vi "Read IBW File.vi"(8 "error in (no error)":errorcluster, 10 "Basename":string, 11 "Path":path) -> (0 "error out":errorcluster, 2 "Notes LUT":variant, 3 "IMAQ":T1[](array[plugin-control]))   [LabVIEW 2019]
uses:
  <vilib>/vision/NI_Vision_Development_Module.lvlib
  <vilib>/Utility/error.llb/whitespace.ctl
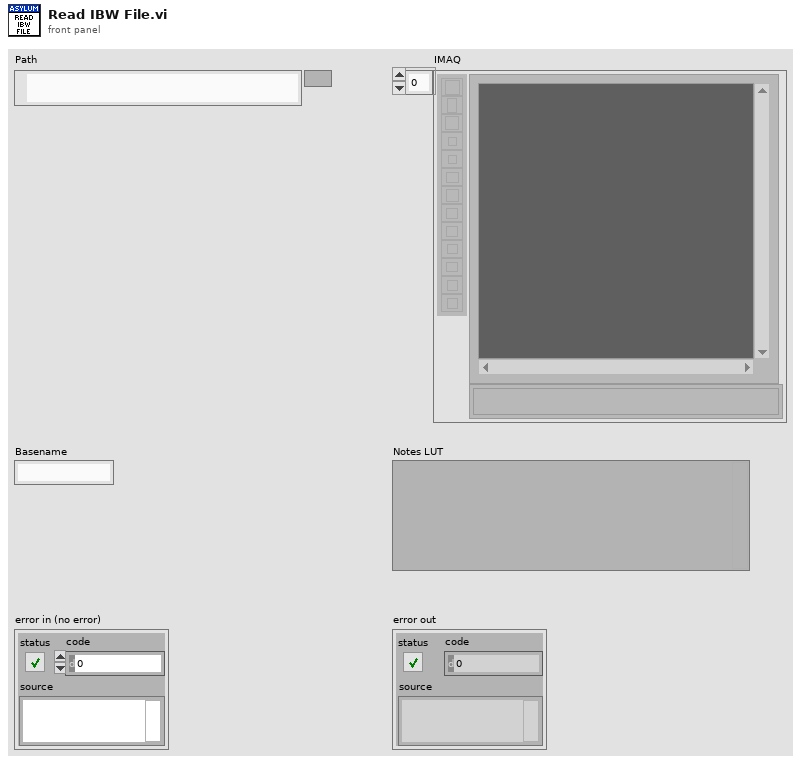
[diagram p1: front panel]
types:
  T1 = typedef "IMAQ Image.ctl" = refnum<image>
  T2 = enum32{"Invalid", "Standard", "Closed", "Hidden", "Minimized", "Maximized"}
  T3 = enum32{"invalid app kind", "Development System", "Run Time System", "Student Edition", "Embedded LabVIEW", "Evaluation", "Custom"}
  T4 = enum16{"big-endian, network order", "native, host order", "little-endian"}
  T5 = cluster{"Core":cluster{"Current VI Reference":refnum<vi>, "Close Panel on Exit?":bool}, "Binary":string, "wfmSize":i32, "noteSize":i32, "nDim":i32[], "wData":sgl[], "Shaped wData":sgl[][][], "Notes":string}
  T6 = cluster{"Current VI Reference":refnum<vi>, "Close Panel on Exit?":bool}
  T7 = typedef "Image Type" = u32
  T8 = typedef "whitespace.ctl" = u16
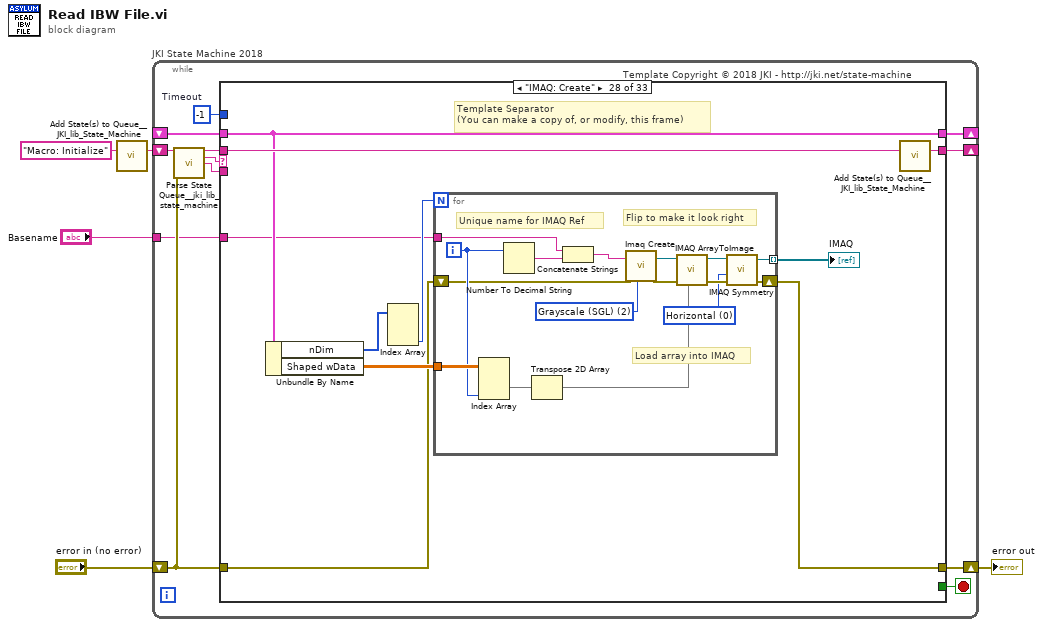
[diagram p0: block diagram]
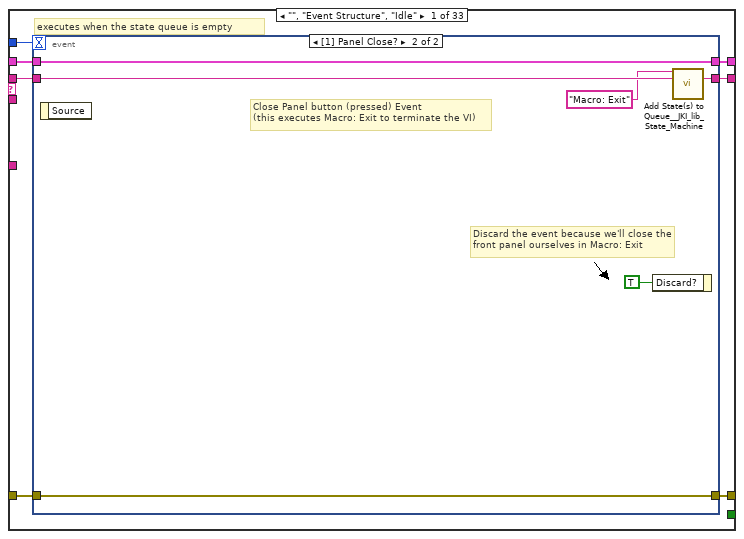
[diagram p2: hidden frame]
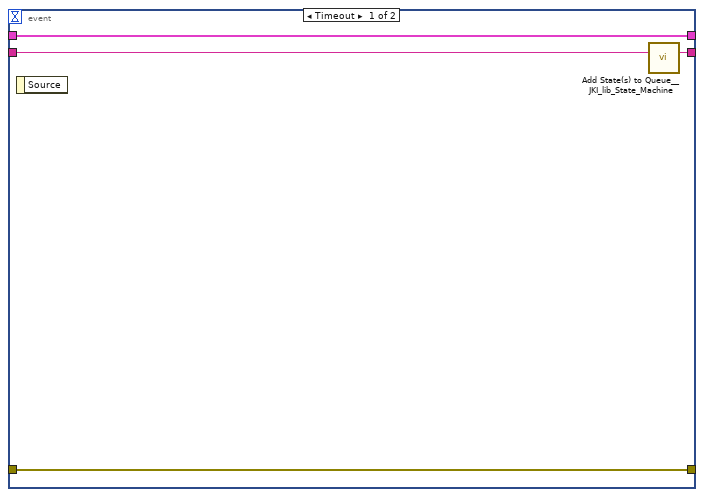
[diagram p3: hidden frame]
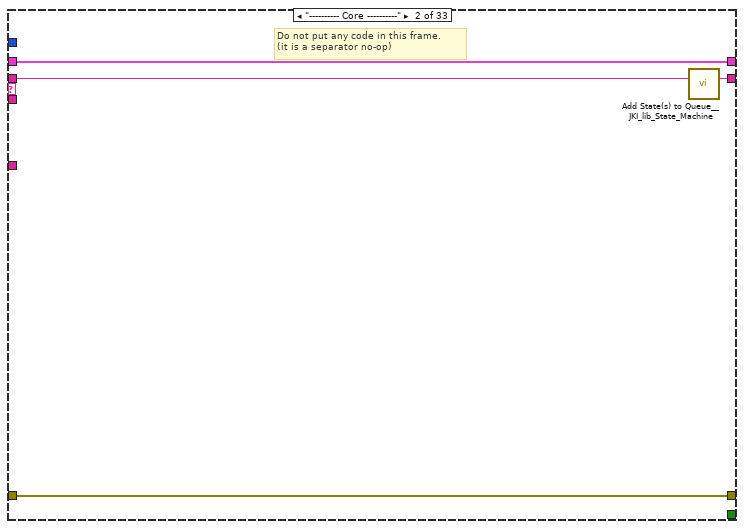
[diagram p4: hidden frame]
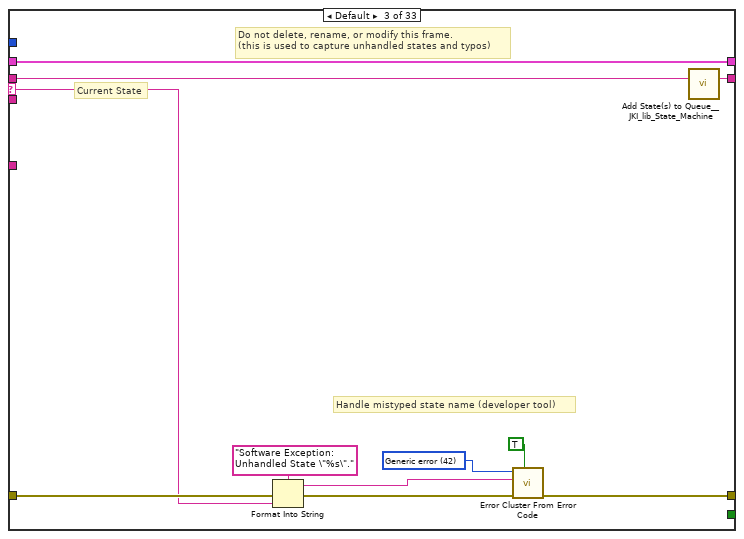
[diagram p5: hidden frame]
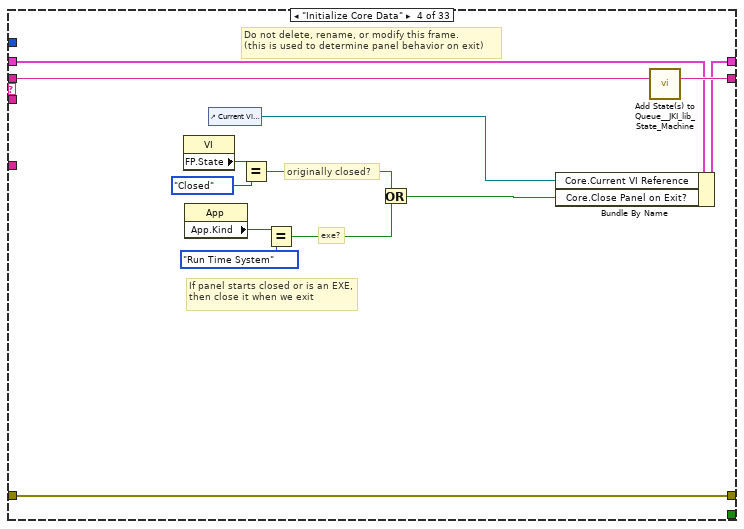
[diagram p6: hidden frame]
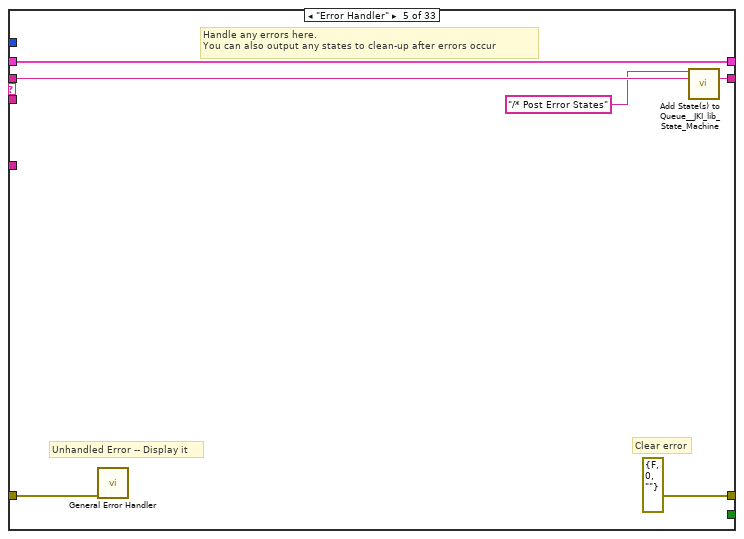
[diagram p7: hidden frame]
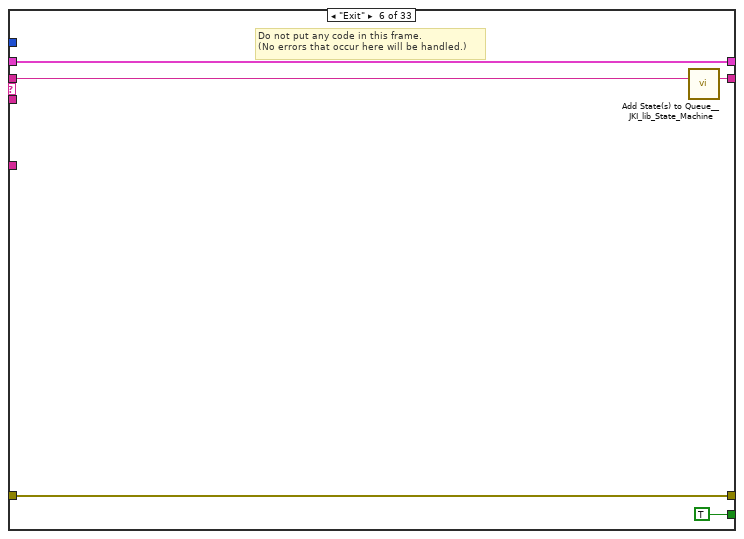
[diagram p8: hidden frame]
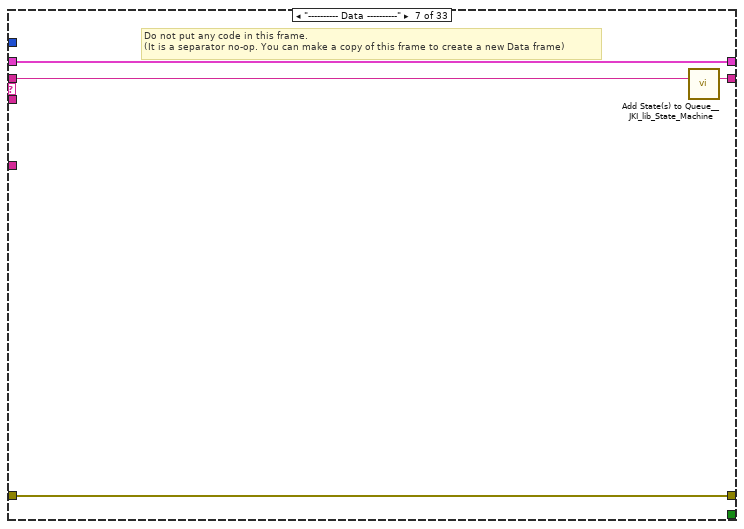
[diagram p9: hidden frame]
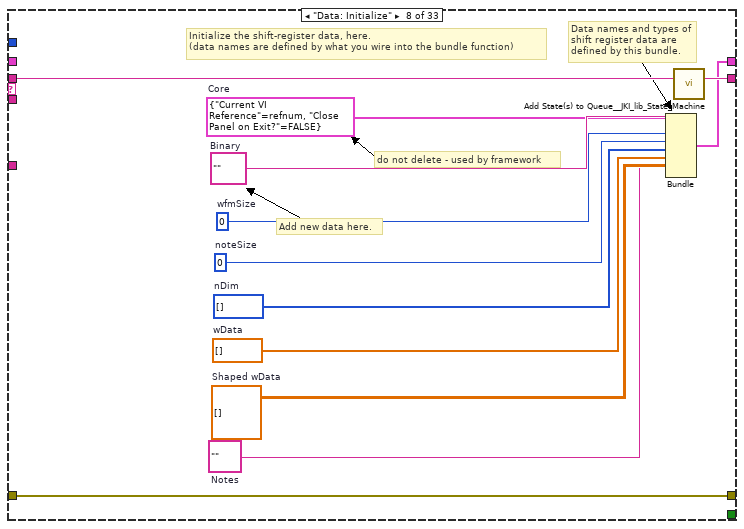
[diagram p10: hidden frame]
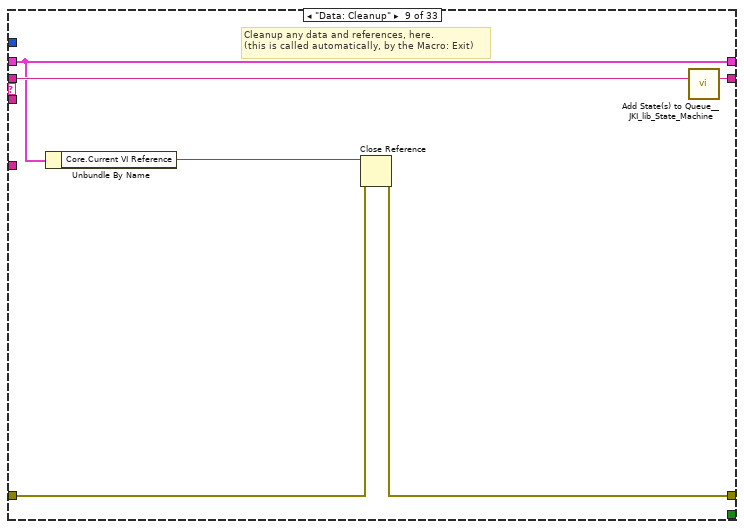
[diagram p11: hidden frame]
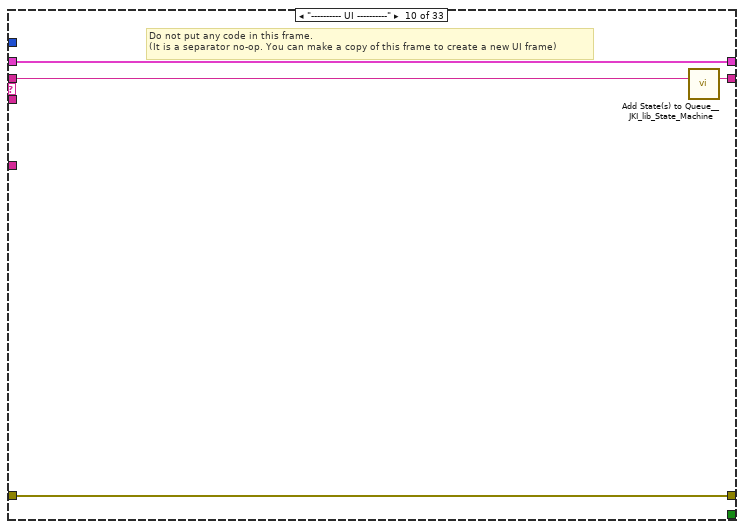
[diagram p12: hidden frame]
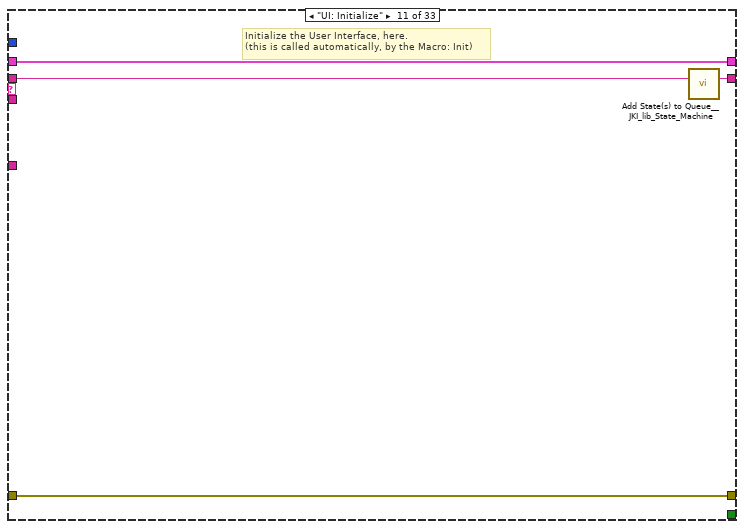
[diagram p13: hidden frame]
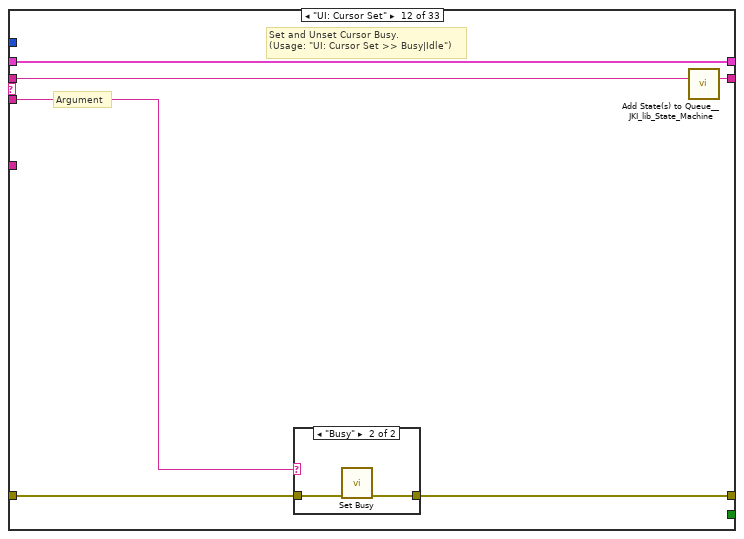
[diagram p14: hidden frame]
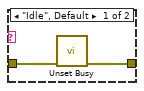
[diagram p15: hidden frame]
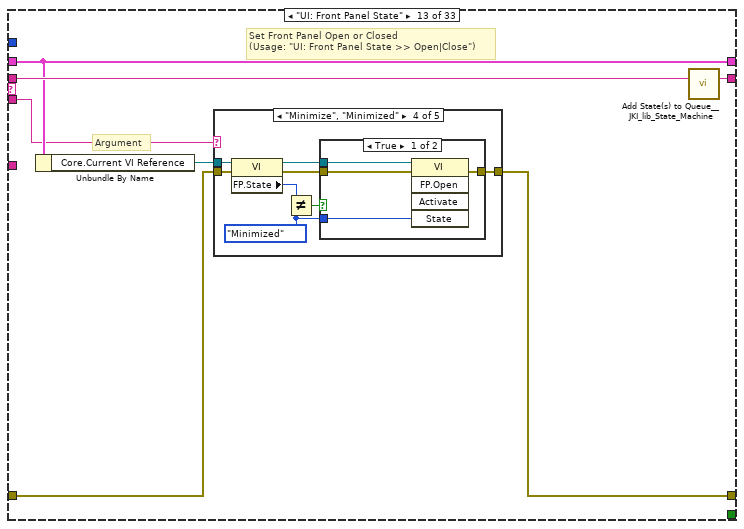
[diagram p16: hidden frame]
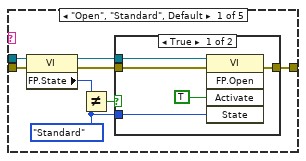
[diagram p17: hidden frame]
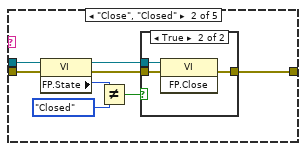
[diagram p19: hidden frame]
diagram:
  n1 = call <vilib>:"Add State(s) to Queue__JKI_lib_State_Machine.vi"("State(s) in (\"\")"="Macro: Initialize") -> ("States Out"=w5:string)  [unwired: 14 in]
  n2 = while "JKI State Machine 2018" {
    shift-right: [w10] -> _
    shift-left: _ -> [w9]
    shift-right: [w13] -> w3
    shift-left: "error in (no error)" -> [w7]
    shift-right: [w12] -> _
    shift-left: w5 -> [w14]
    tunnel: "Basename" -> [w6]
    stop <- w11 stop-if-true
    w8 = -1  # Timeout
    # "Template Copyright © 2018 JKI - http://jki.net/state-machine"
    n3 = call <vilib>:"Parse State Queue__jki_lib_state_machine.vi"("State Queue"=w14, "Error In (no error)"=w7) -> ("Remaining States"=w16:string, "Current State"=w17:string, "Arguments"=w15:string)  [unwired: 11 in]
    n4 = case shown="\"IMAQ: Create\"" w17 {
      selector: w17 -> [_ _ w39 _ _ _ _ _ _ _ _ _ _ _ _ _ _ _ _ _ _ _ _ _ _ _ _ _ _ _ _ _ _]
      tunnel: w16 -> [w24 w38 w43 w62 w68 w73 w77 w89 w95 w99 w103 w109 w120 w189 w194 w199 w209 w213 w221 w225 w238 w251 w264 w285 w300 w336 w340 w350 w370 w380 w403 w407 w411]
      tunnel: w15 -> [_ _ _ _ _ _ _ _ _ _ _ w104 w114 _ _ _ _ _ _ _ _ _ _ _ _ _ _ _ _ _ _ _ _]
      tunnel: w9 -> [w22 w35 w41 w55 w65 w71 w74 _ w90 w96 w101 w107 w116 w186 w191 w196 w206 w210 w217 w222 w227 w240 w254 w275 w292 w327 w337 w343 w367 w378 w400 w404 w408]
      tunnel: [w21 w36 w45 w59 errorcluster {"status"=FALSE, "code"=0, "source"=""} ("error out") w70 w75 w86 w91 w97 w100 w105 w117 w187 w192 w197 w207 w211 w215 w223 w236 w249 w262 w266 w298 w334 w338 w344 w368 w372 w401 w405 w409] -> w13
      tunnel: w7 -> [w20 w36 w44 w59 w64 w70 w75 w86 w92 w97 w100 w106 w118 w187 w192 w197 w207 w211 w214 w223 w236 w249 w262 w267 w298 w334 w338 w345 w368 w371 w401 w405 w409]
      tunnel: [w23 w37 w42 w61 w67 w72 w76 w88 w94 w98 w102 w108 w119 w188 w193 w198 w208 w212 w220 w224 w237 w250 w263 w284 w299 w335 w339 w349 w369 w379 w402 w406 w410] -> w12
      tunnel: [_ _ _ _ _ TRUE _ _ _ _ _ _ _ _ _ _ _ _ _ _ _ _ _ _ _ _ _ _ _ _ _ _ _] -> w11
      tunnel: [w19 w35 w41 w60 w65 w71 w74 w87 w90 w96 w101 w107 w116 w186 w191 w196 w206 w210 w218 w222 w228 w241 w255 w276 w293 w328 w337 w343 w367 w378 w400 w404 w408] -> w10
      tunnel: w8 -> [w18 _ _ _ _ _ _ _ _ _ _ _ _ _ _ _ _ _ _ _ _ _ _ _ _ _ _ _ _ _ _ _ _]
      tunnel: w6 -> [_ _ _ _ _ _ _ _ _ _ _ _ _ _ _ _ _ _ _ _ _ _ _ _ _ _ _ w342 _ _ _ _ _]
      frame "", "Event Structure", "Idle" {
        # "executes when the state queue is empty"
        n5 = event shown="[1] Panel Close?" {
          selector: _ -> [_ _]
          dyn-events: _ -> [_ _]
          timeout: w18 -> [_ _]
          tunnel: w24 -> [w28 w34]
          tunnel: [w27 w33] -> w23
          tunnel: w22 -> [w25 w31]
          tunnel: [w26 w32] -> w21
          tunnel: w20 -> [w26 w32]
          tunnel: [w25 w31] -> w19
          event Timeout {
            n6 = event-data() -> ()  [unwired: 1 in, 1 out]
            n7 = call <vilib>:"Add State(s) to Queue__JKI_lib_State_Machine.vi"("State(s) in (\"\")"=w28) -> ("States Out"=w27:string)  [unwired: 14 in]
          }
          event Panel Close? {
            # "Discard the event because we'll close the front panel ourselves in Macro: Exit"
            # "Close Panel button (pressed) Event\n(this executes Macro: Exit to terminate the VI)"
            n8 = event-data() -> ()  [unwired: 1 in, 1 out]
            n9 = event-data ("Event Filter Node")("Discard?"=TRUE) -> ()  [unwired: 1 in, 1 out]
            n10 = call <vilib>:"Add State(s) to Queue__JKI_lib_State_Machine.vi"("State(s) in Front (\"\")"="Macro: Exit", "State(s) in (\"\")"=w34) -> ("States Out"=w33:string)  [unwired: 13 in]
          }
        }
      }
      frame "---------- Core ----------" {
        # "Do not put any code in this frame.\n(it is a separator no-op)"
        n11 = call <vilib>:"Add State(s) to Queue__JKI_lib_State_Machine.vi"("State(s) in (\"\")"=w38) -> ("States Out"=w37:string)  [unwired: 14 in]
      }
      frame Default {
        w48 = 42 items=["No error", "Argument error", "Memory is full", "Out of zone", "End of file", "File already open", "Generic file I/O error", "File not found", "File permission error", "Disk is full", "Duplicate path", "Too many files open", "System feature not enabled", "Resource file not found", "Cannot add resource", "Resource not found", "Image not found", "Image memory error", "Pen does not exist", "Config type invalid", "Config token not found", "Config parse error", "Config memory error", "Bad external code format", "Bad external code offset", "External code not present", "Null window", "Destroy window error", "Null menu", "Print aborted", "Bad print record", "Print driver error", "Windows error during printing", "Memory error during printing", "Print dialog error", "Generic print error", "Invalid device refnum", "Device not found", "Device parameter error", "Device unit error", "Cannot open device", "Device call aborted", "Generic error", "Cancelled by user", "Object ID too low", "Object ID too high", "Object not in heap", "Unknown heap", "Unknown object (invalid DefProc)", "Unknown object (DefProc not in table)", "Message out of range", "Invalid (null) method", "Unknown message", "Manager call not supported", "Bad address", "Network operation in progress", "Network operation timed out", "Connection is busy", "Network attribute not supported", "Network error", "Address in use", "System out of memory", "Connection aborted", "Connection refused", "Not connected", "Already connected", "Connection closed", "Initialization error (interapplication manager)", "Bad occurrence", "Wait on unbound occurrence handler", "Occurrence queue overflow", "Datalog type conflict", "Unused", "Unrecognized type (interapplication manager)", "Memory corrupt", "Failed to make temporary DLL", "Old CIN version", "Drag socket not found", "Failed to load drop-object", "Failed to register OLE object", "Failed to release OLE object", "Format specifier type mismatch", "Unknown format specifier", "Too few format specifiers", "Too many format specifiers", "Scan failed", "Newer CIN version", "Error converting to variant", "Runtime menu error", "Password tampered", "Variant attribute not found", "Incompatible variant data type", "Event data is not available", "Event Store is not present", "Occurrence is not found", "Event Queue is not created", "Event info is not available", "Refnum passed is NULL", "Error retrieving Class GUID", "Error retrieving CoClass GUID", "Error retrieving TypeLib GUID.", "Bad built application magic bytes.", "Specific driver is different from the specific driver associated with the Logical Name.", "There is no session opened to the class driver.", "Max Error", "MAX - Error with config objects", "MAX - Error loading configuration", "MAX - Group not supported"]
        # "Current State"
        # "Do not delete, rename, or modify this frame.\n(this is used to capture unhandled states and typos)"
        # "Handle mistyped state name (developer tool)"
        n12 = Format Into String(format string="Software Exception: Unhandled State \"%s\"." ("message"), error in=w44, w39) -> (resulting string=w47:string, error out=w46:errorcluster)  [unwired: 1 in]
        n13 = call <vilib>:"Error Cluster From Error Code.vi"("show call chain? (False)"=TRUE, "error in (no error)"=w46, "error message (\"\")"=w47, "error code (0)"=w48) -> ("error out"=w45:errorcluster)  [unwired: 5 in]
        n14 = call <vilib>:"Add State(s) to Queue__JKI_lib_State_Machine.vi"("State(s) in (\"\")"=w43) -> ("States Out"=w42:string)  [unwired: 14 in]
      }
      frame "Initialize Core Data" {
        # "Do not delete, rename, or modify this frame.\n(this is used to determine panel behavior on exit)"
        # "originally closed?"
        # "exe?"
        # "If panel starts closed or is an EXE, then close it when we exit"
        n15 = property on="Property Node" class="VI"() -> ("FP.State"=w52:T2)  [unwired: 2 in, 2 out]
        n16 = property on="Property Node" class="App"() -> ("App.Kind"=w58:T3)  [unwired: 2 in, 2 out]
        n17 = control-ref of="Current VI Reference"() -> (w53:refnum<vi>)
        n18 = Equal?(x=w52, y=T2."Closed" ("Front Panel Window:State")) -> (x = y?=w50:bool)
        n19 = Equal?(x=w58, y=T3."Run Time System" ("Application:Kind")) -> (x = y?=w56:bool)
        n20 = Or(x=w50, y=w56) -> (x .or. y?=w54:bool)
        n21 = Bundle By Name(cluster=w55, "Core.Current VI Reference"=w53, "Core.Close Panel on Exit?"=w54) -> (w60:T5)
        n22 = call <vilib>:"Add State(s) to Queue__JKI_lib_State_Machine.vi"("State(s) in (\"\")"=w62) -> ("States Out"=w61:string)  [unwired: 14 in]
      }
      frame "Error Handler" {
        # "Unhandled Error -- Display it"
        # "Handle any errors here.\nYou can also output any states to clean-up after errors occur"
        # "Clear error"
        n23 = call <vilib>:"General Error Handler.vi"("error in (no error)"=w64) -> ()  [unwired: 10 in, 5 out]
        n24 = call <vilib>:"Add State(s) to Queue__JKI_lib_State_Machine.vi"("State(s) in Front (\"\")"="/* Post Error States", "State(s) in (\"\")"=w68) -> ("States Out"=w67:string)  [unwired: 13 in]
      }
      frame "Exit" {
        # "Do not put any code in this frame.\n(No errors that occur here will be handled.)"
        n25 = call <vilib>:"Add State(s) to Queue__JKI_lib_State_Machine.vi"("State(s) in (\"\")"=w73) -> ("States Out"=w72:string)  [unwired: 14 in]
      }
      frame "---------- Data ----------" {
        # "Do not put any code in this frame.\n(It is a separator no-op. You can make a copy of this frame to create a new Data frame)"
        n26 = call <vilib>:"Add State(s) to Queue__JKI_lib_State_Machine.vi"("State(s) in (\"\")"=w77) -> ("States Out"=w76:string)  [unwired: 14 in]
      }
      frame "Data: Initialize" {
        w78 = ""  # Notes
        w79 = sgl[][][] []  # Shaped wData
        w80 = sgl[] []  # wData
        w81 = i32[] []  # nDim
        w82 = 0  # noteSize
        w83 = 0  # wfmSize
        w84 = T6 {"Current VI Reference"=refnum, "Close Panel on Exit?"=FALSE}  # Core
        w85 = ""  # Binary
        # "do not delete - used by framework"
        # "Add new data here."
        # "Data names and types of shift register data are defined by this bundle."
        # "Initialize the shift-register data, here.\n(data names are defined by what you wire into the bundle function)"
        n27 = Bundle("Core"=w84, "Binary"=w85, "wfmSize"=w83, "noteSize"=w82, "nDim"=w81, "wData"=w80, "Shaped wData"=w79, "Notes"=w78) -> (w87:T5)  [unwired: 1 in]
        n28 = call <vilib>:"Add State(s) to Queue__JKI_lib_State_Machine.vi"("State(s) in (\"\")"=w89) -> ("States Out"=w88:string)  [unwired: 14 in]
      }
      frame "Data: Cleanup" {
        # "Cleanup any data and references, here.\n(this is called automatically, by the Macro: Exit)"
        n29 = Unbundle By Name(w90) -> ("Core.Current VI Reference"=w93:refnum<vi>)
        n30 = Close Reference(reference=w93, error in (no error)=w92) -> (error out=w91:errorcluster)
        n31 = call <vilib>:"Add State(s) to Queue__JKI_lib_State_Machine.vi"("State(s) in (\"\")"=w95) -> ("States Out"=w94:string)  [unwired: 14 in]
      }
      frame "---------- UI ----------" {
        # "Do not put any code in this frame.\n(It is a separator no-op. You can make a copy of this frame to create a new UI frame)"
        n32 = call <vilib>:"Add State(s) to Queue__JKI_lib_State_Machine.vi"("State(s) in (\"\")"=w99) -> ("States Out"=w98:string)  [unwired: 14 in]
      }
      frame "UI: Initialize" {
        # "Initialize the User Interface, here.\n(this is called automatically, by the Macro: Init)"
        n33 = call <vilib>:"Add State(s) to Queue__JKI_lib_State_Machine.vi"("State(s) in (\"\")"=w103) -> ("States Out"=w102:string)  [unwired: 14 in]
      }
      frame "UI: Cursor Set" {
        # "Argument"
        # "Set and Unset Cursor Busy.\n(Usage: \"UI: Cursor Set >> Busy|Idle\")"
        n34 = case shown="\"Busy\"" w104 {
          tunnel: w106 -> [w111 w113]
          tunnel: [w110 w112] -> w105
          frame "Idle", Default {
            n35 = call <vilib>:"Unset Busy.vi"("error in (no error)"=w111) -> ("error out"=w110:errorcluster)  [unwired: 10 in]
          }
          frame "Busy" {
            n36 = call <vilib>:"Set Busy.vi"("error in (no error)"=w113) -> ("error out"=w112:errorcluster)  [unwired: 9 in, 1 out]
          }
        }
        n37 = call <vilib>:"Add State(s) to Queue__JKI_lib_State_Machine.vi"("State(s) in (\"\")"=w109) -> ("States Out"=w108:string)  [unwired: 14 in]
      }
      frame "UI: Front Panel State" {
        # "Argument"
        # "Set Front Panel Open or Closed\n(Usage: \"UI: Front Panel State >> Open|Close\")"
        n38 = Unbundle By Name(w116) -> ("Core.Current VI Reference"=w115:refnum<vi>)
        n39 = case shown="\"Minimize\", \"Minimized\"" w114 {
          tunnel: w118 -> [w126 w141 w152 w165 w178]
          tunnel: [w128 w142 w154 w167 w180] -> w117
          tunnel: w115 -> [w127 w139 w153 w166 w179]
          frame "Open", "Standard", Default {
            w121 = T2."Standard" ("State")
            n40 = property on="Property Node" class="VI"(reference=w127, error in=w126) -> (reference out=w124:refnum<vi>, error out=w125:errorcluster, "FP.State"=w123:T2)
            n41 = Not Equal?(x=w123, y=w121) -> (x != y?=w122:bool)
            n42 = case shown="True" w122 {
              tunnel: [w132 w134] -> w128
              tunnel: w125 -> [w131 w134]
              tunnel: w124 -> [w130 _]
              tunnel: w121 -> [w129 _]
              frame True {
                n43 = invoke on="Invoke Node" class="VI" method="FP.Open"(reference=w130, error in=w131, "Activate"=TRUE, "State"=w129) -> (error out=w132:errorcluster)  [unwired: 1 in, 4 out]
              }
              frame False {
              }
            }
          }
          frame "Close", "Closed" {
            n44 = property on="Property Node" class="VI"(reference=w139, error in=w141) -> (reference out=w138:refnum<vi>, error out=w140:errorcluster, "FP.State"=w136:T2)
            n45 = Not Equal?(x=w136, y=T2."Closed" ("Front Panel Window:State")) -> (x != y?=w135:bool)
            n46 = case shown="True" w135 {
              tunnel: [w143 w146] -> w142
              tunnel: w140 -> [w143 w145]
              tunnel: w138 -> [_ w144]
              frame False {
              }
              frame True {
                n47 = invoke on="Invoke Node" class="VI" method="FP.Close"(reference=w144, error in=w145) -> (error out=w146:errorcluster)  [unwired: 1 in, 2 out]
              }
            }
          }
          frame "Hidden", "Hide" {
            w147 = T2."Hidden" ("State")
            n48 = property on="Property Node" class="VI"(reference=w153, error in=w152) -> (reference out=w150:refnum<vi>, error out=w151:errorcluster, "FP.State"=w149:T2)
            n49 = Not Equal?(x=w149, y=w147) -> (x != y?=w148:bool)
            n50 = case shown="True" w148 {
              tunnel: [w158 w159] -> w154
              tunnel: w151 -> [w157 w159]
              tunnel: w150 -> [w156 _]
              tunnel: w147 -> [w155 _]
              frame True {
                n51 = invoke on="Invoke Node" class="VI" method="FP.Open"(reference=w156, error in=w157, "State"=w155) -> (error out=w158:errorcluster)  [unwired: 2 in, 4 out]
              }
              frame False {
              }
            }
          }
          frame "Minimize", "Minimized" {
            w160 = T2."Minimized" ("State")
            n52 = property on="Property Node" class="VI"(reference=w166, error in=w165) -> (reference out=w163:refnum<vi>, error out=w164:errorcluster, "FP.State"=w162:T2)
            n53 = Not Equal?(x=w162, y=w160) -> (x != y?=w161:bool)
            n54 = case shown="True" w161 {
              tunnel: [w171 w172] -> w167
              tunnel: w164 -> [w170 w172]
              tunnel: w163 -> [w169 _]
              tunnel: w160 -> [w168 _]
              frame True {
                n55 = invoke on="Invoke Node" class="VI" method="FP.Open"(reference=w169, error in=w170, "State"=w168) -> (error out=w171:errorcluster)  [unwired: 2 in, 4 out]
              }
              frame False {
              }
            }
          }
          frame "Maximize", "Maximized" {
            w173 = T2."Maximized" ("State")
            n56 = property on="Property Node" class="VI"(reference=w179, error in=w178) -> (reference out=w176:refnum<vi>, error out=w177:errorcluster, "FP.State"=w175:T2)
            n57 = Not Equal?(x=w175, y=w173) -> (x != y?=w174:bool)
            n58 = case shown="True" w174 {
              tunnel: [w184 w185] -> w180
              tunnel: w177 -> [w183 w185]
              tunnel: w176 -> [w182 _]
              tunnel: w173 -> [w181 _]
              frame True {
                n59 = invoke on="Invoke Node" class="VI" method="FP.Open"(reference=w182, error in=w183, "State"=w181) -> (error out=w184:errorcluster)  [unwired: 2 in, 4 out]
              }
              frame False {
              }
            }
          }
        }
        n60 = call <vilib>:"Add State(s) to Queue__JKI_lib_State_Machine.vi"("State(s) in (\"\")"=w120) -> ("States Out"=w119:string)  [unwired: 14 in]
      }
      frame "---------- Macro ----------" {
        # "Backups in case Directory State gets deleted on accident since those are never called"
        # "Length|Index|typedef struct BinHeader5 {\n     2|    0|\tshort version;\t\t\t\t\t\t          // Version number for backwards compatibility.\n     2|    2|\tshort checksum;\t\t\t\t\t\t         // Checksum over this header and the wave header.\n     4|    4|\tlong wfmSize;\t\t\t\t\t\t           // The size of the WaveHeader5 data structure plus the wave data.\n     4|    8|\tlong formulaSize;\t\t\t\t\t        // The size of the dependency formula, if any.\n     4|   12|\tlong noteSize;\t\t\t\t\t\t          // The size of the note text.\n     4|   16|\tlong dataEUnitsSize;\t\t\t\t      // The size of optional extended data units.\n    16|   20|\tlong dimEUnitsSize[MAXDIMS];\t\t// The size of optional extended dimension units.\n    16|   36|\tlong dimLabelsSize[MAXDIMS];\t\t// The size of optional dimension labels.\n     4|   52|\tlong sIndicesSize;\t\t\t\t\t       // The size of string indicies if this is a text wave.\n     4|   56|\tlong optionsSize1;\t\t\t\t\t       // Reserved. Write zero. Ignore on read.\n     4|   60|\tlong optionsSize2;\t\t\t\t\t       // Reserved. Write zero. Ignore on read.\n      |   64|} BinHeader5;"
        # "Length|Index|struct WaveHeader5 {\n     4|   64|\tstruct WaveHeader5 **next;\t\t\t  // link to next wave in linked list.\n     4|   68|\tunsigned long creationDate;\t\t \t// DateTime of creation.\n     4|   72|\tunsigned long modDate;\t\t\t\t     // DateTime of last modification.\n     4|   76|\tlong npnts;\t\t\t\t\t\t\t             // Total number of points (multiply dimensions up to first zero).\n     2|   80|\tshort type;\t\t\t\t\t\t\t             // See types (e.g. NT_FP64) above. Zero for text waves.\n     2|   82|\tshort dLock;\t\t\t\t\t\t             // Reserved. Write zero. Ignore on read.\n     6|   84|\tchar whpad1[6];\t\t\t\t\t\t          // Reserved. Write zero. Ignore on read.\n     2|   90|\tshort whVersion;\t\t\t\t\t          // Write 1. Ignore on read.\n    32|   92|\tchar bname[MAX_WAVE_NAME5+1];\t\t// Name of wave plus trailing null.\n     4|  124|\tlong whpad2;\t\t\t\t\t\t             // Reserved. Write zero. Ignore on read.\n     4|  128|\tstruct DataFolder **dFolder;\t\t // Used in memory only. Write zero. Ignore on read.\n      |     |\t// Dimensioning info. [0] == rows, [1] == cols etc\n    16|  132|\tlong nDim[MAXDIMS];\t\t\t\t\t       // Number of of items in a dimension -- 0 means no data.\n    32|  148|\tdouble sfA[MAXDIMS];\t\t\t\t       // Index value for element e of dimension d = sfA[d]*e + sfB[d].\n    32|  180|\tdouble sfB[MAXDIMS];\n      |     |\t// SI units\n     4|  212|\tchar dataUnits[MAX_UNIT_CHARS+1];\t\t\t      // Natural data units go here - null if none.\n    16|  216|\tchar dimUnits[MAXDIMS][MAX_UNIT_CHARS+1];\t// Natural dimension units go here - null if none.\n     2|  232|\tshort fsValid;\t\t\t\t\t\t                      // TRUE if full scale values have meaning.\n     2|  234|\tshort whpad3;\t\t\t\t\t\t                       // Reserved. Write zero. Ignore on read.\n    16|  236|\tdouble topFullScale,botFullScale;\t        // The max and max full scale value for wave.\n     4|  252|\tHandle dataEUnits;\t\t\t\t\t                   // Used in memory only. Write zero. Ignore on read.\n    16|  256|\tHandle dimEUnits[MAXDIMS];\t\t\t             // Used in memory only. Write zero. Ignore on read.\n    16|  272|\tHandle dimLabels[MAXDIMS];\t\t\t             // Used in memory only. Write zero. Ignore on read.\n     4|  288|\tHandle waveNoteH;\t\t\t\t\t                    // Used in memory only. Write zero. Ignore on read.\n    64|  292|\tlong whUnused[16];\t\t\t\t\t                   // Reserved. Write zero. Ignore on read.\n      |     |\t// The following stuff is considered private to Igor.\n     2|  356|\tshort aModified;\t\t\t\t\t                     // Used in memory only. Write zero. Ignore on read.\n     2|  358|\tshort wModified;\t\t\t\t\t                     // Used in memory only. Write zero. Ignore on read.\n     2|  360|\tshort swModified;\t\t\t\t\t                    // Used in memory only. Write zero. Ignore on read.\n     1|  362|\tchar useBits;\t\t\t\t\t\t                       // Used in memory only. Write zero. Ignore on read.\n     1|  363|\tchar kindBits;\t\t\t\t\t\t                      // Reserved. Write zero. Ignore on read.\n     4|  364|\tvoid **formula;\t\t\t\t\t\t                     // Used in memory only. Write zero. Ignore on read.\n     4|  368|\tlong depID;\t\t\t\t\t\t\t                        // Used in memory only. Write zero. Ignore on read.\n     2|  372|\tshort whpad4;\t\t\t\t\t\t                       // Reserved. Write zero. Ignore on read.\n     2|  374|\tshort srcFldr;\t\t\t\t\t\t                      // Used in memory only. Write zero. Ignore on read.\n     4|  376|\tHandle fileName;\t\t\t\t\t                     // Used in memory only. Write zero. Ignore on read.\n     4|  380|\tlong **sIndices;\t\t\t\t\t                     // Used in memory only. Write zero. Ignore on read.\n     4|  384|\tfloat wData[1];\t\t\t\t\t\t                     // The start of the array of data. Must be 64 bit aligned.\n      |  388|};"
        # "Do not put any code in this frame.\n(It is a separator no-op. You can make a copy of this frame to create a new Macro frame)"
        n61 = call <vilib>:"Add State(s) to Queue__JKI_lib_State_Machine.vi"("State(s) in (\"\")"=w189) -> ("States Out"=w188:string)  [unwired: 14 in]
      }
      frame "Macro: Initialize" {
        # "Initialization Macro\n(This is called once, when the VI starts)"
        n62 = call <vilib>:"Add State(s) to Queue__JKI_lib_State_Machine.vi"("State(s) in Front (\"\")"="Data: Initialize\nInitialize Core Data\n//UI: Initialize\n//UI: Front Panel State >> Open\n\nMacro: Parse IBW\n\nMacro: Exit", "State(s) in (\"\")"=w194) -> ("States Out"=w193:string)  [unwired: 13 in]
      }
      frame "Macro: Parse IBW" {
        # "Parse IBW Macro\n(This is called once, when the VI starts)"
        n63 = call <vilib>:"Add State(s) to Queue__JKI_lib_State_Machine.vi"("State(s) in Front (\"\")"="File: Read\nParse: wfmSize\nParse: noteSize\nParse: nDim\nParse: wData\nParse: Shape wData\nParse: Notes\nIMAQ: Create\nNotes: Create LUT", "State(s) in (\"\")"=w199) -> ("States Out"=w198:string)  [unwired: 13 in]
      }
      frame "Macro: Exit" {
        # "Exit Macro\n(This is called once, when the VI exits)"
        n64 = Unbundle By Name(w206) -> ("Core.Close Panel on Exit?"=w205:bool)
        n65 = Select(t="UI: Front Panel State >> Close", s=w205, f="" ("Empty String Constant")) -> (s? t:f=w202:string)
        n66 = call <vilib>:"Add State(s) to Queue__JKI_lib_State_Machine.vi"("State(s) in (\"\")"=w202, "State(s) at Back (\"\")"="Data: Cleanup\nExit") -> ("States Out"=w200:string)  [unwired: 13 in]
        n67 = call <vilib>:"Add State(s) to Queue__JKI_lib_State_Machine.vi"("State(s) in Front (\"\")"=w200, "State(s) in (\"\")"=w209) -> ("States Out"=w208:string)  [unwired: 13 in]
      }
      frame "---------- File ----------" {
        # "Template Separator\n(You can make a copy of, or modify, this frame)"
        n68 = call <vilib>:"Add State(s) to Queue__JKI_lib_State_Machine.vi"("State(s) in (\"\")"=w213) -> ("States Out"=w212:string)  [unwired: 14 in]
      }
      frame "File: Read" {
        # "Ensure that Convert EOL? is set to False."
        # "File: Read\n(read characters from file)"
        n69 = Read from Text File(file (use dialog)="Path", error in=w214) -> (text=w216:string, error out=w215:errorcluster)  [unwired: 2 in, 2 out]
        n70 = Bundle By Name(cluster=w217, "Binary"=w216) -> (w218:T5)
        n71 = call <vilib>:"Add State(s) to Queue__JKI_lib_State_Machine.vi"("State(s) in (\"\")"=w221) -> ("States Out"=w220:string)  [unwired: 14 in]
      }
      frame "---------- Parse ----------" {
        # "Template Separator\n(You can make a copy of, or modify, this frame)"
        n72 = call <vilib>:"Add State(s) to Queue__JKI_lib_State_Machine.vi"("State(s) in (\"\")"=w225) -> ("States Out"=w224:string)  [unwired: 14 in]
      }
      frame "Parse: wfmSize" {
        # "From Big Endian to Little Endian"
        # "Convert to integer"
        # "Location: See Directory"
        # "Parse: wfmSize\n(*)"
        n73 = Unbundle By Name(w227) -> ("Binary"=w235:string)
        n74 = String Subset(string=w235, offset (0)=4, length (rest)=4 ("length (rest)")) -> (substring=w232:string)
        n75 = Type Cast(type=0, x=w232) -> (*(type *) &x=w230:i32)
        n76 = Swap Bytes(anything=w230) -> (byte swapped=w231:i32)
        n77 = Swap Words(1:w231) -> (0:w226:i32)
        n78 = Bundle By Name(cluster=w227, "wfmSize"=w226) -> (w228:T5)
        n79 = call <vilib>:"Add State(s) to Queue__JKI_lib_State_Machine.vi"("State(s) in (\"\")"=w238) -> ("States Out"=w237:string)  [unwired: 14 in]
      }
      frame "Parse: noteSize" {
        # "From Big Endian to Little Endian"
        # "Convert to integer"
        # "Location: See Directory"
        # "Parse: noteSize\n(*)"
        n80 = Unbundle By Name(w240) -> ("Binary"=w248:string)
        n81 = String Subset(string=w248, offset (0)=12, length (rest)=4 ("length (rest)")) -> (substring=w245:string)
        n82 = Type Cast(type=0, x=w245) -> (*(type *) &x=w243:i32)
        n83 = Swap Bytes(anything=w243) -> (byte swapped=w244:i32)
        n84 = Swap Words(1:w244) -> (0:w239:i32)
        n85 = Bundle By Name(cluster=w240, "noteSize"=w239) -> (w241:T5)
        n86 = call <vilib>:"Add State(s) to Queue__JKI_lib_State_Machine.vi"("State(s) in (\"\")"=w251) -> ("States Out"=w250:string)  [unwired: 14 in]
      }
      frame "Parse: nDim" {
        # "From Big Endian to Little Endian"
        # "Convert to integer"
        # "Location: See Directory"
        # "Parse: nDim\n(*)"
        n87 = Unbundle By Name(w254) -> ("Binary"=w256:string)
        n88 = String Subset(string=w256, offset (0)=132, length (rest)=16 ("length (rest)")) -> (substring=w261:string)
        n89 = Type Cast(type=i32[] [], x=w261) -> (*(type *) &x=w259:i32[])
        n90 = Swap Bytes(anything=w259) -> (byte swapped=w260:i32[])
        n91 = Swap Words(1:w260) -> (0:w253:i32[])
        n92 = Bundle By Name(cluster=w254, "nDim"=w253) -> (w255:T5)
        n93 = call <vilib>:"Add State(s) to Queue__JKI_lib_State_Machine.vi"("State(s) in (\"\")"=w264) -> ("States Out"=w263:string)  [unwired: 14 in]
      }
      frame "Parse: wData" {
        # "Convert from big endian to little endian for SGL"
        # "From the Igor Technical Document:\nwaveDataSize = wfmSize - offsetof(WaveHeader5, wData)\noffset of wData inside of WaveHeader5. This would be 320 (384-64)"
        # "Parse: wData\n(*)"
        n94 = Unbundle By Name(w275) -> ("Binary"=w281:string, "wfmSize"=w283:i32)
        n95 = Subtract(x=w283, y=320) -> (x-y=w279:i32)
        n96 = String Subset(string=w281, offset (0)=384, length (rest)=w279) -> (substring=w278:string)
        n97 = Type Cast(type=sgl[] [], x=w278) -> (*(type *) &x=w274:sgl[])
        n98 = Flatten To String(anything=w274, prepend array or string size? (T)=FALSE, byte order (0:big-endian, network order)=T4."big-endian, network order", error in (no error)=w267) -> (data string=w272:string, error out=w268:errorcluster)  [unwired: 1 out]
        n99 = Unflatten From String(type=w274, binary string=w272, data includes array or string size? (T)=FALSE, byte order (0:big-endian, network order)=T4."little-endian", error in (no error)=w268) -> (value=w273:sgl[], error out=w266:errorcluster)  [unwired: 1 out]
        n100 = Bundle By Name(cluster=w275, "wData"=w273) -> (w276:T5)
        n101 = call <vilib>:"Add State(s) to Queue__JKI_lib_State_Machine.vi"("State(s) in (\"\")"=w285) -> ("States Out"=w284:string)  [unwired: 14 in]
      }
      frame "Parse: Shape wData" {
        # "There are a lot of points\nDont want to duplicate data"
        # "Create array of zeros with dimensions i, j, k\nfor i in nDim[0]:\n     for j in nDim[1]:\n          for k in nDim[2]:\n               replace {zeros[i,j,k]} with wData[i+j+k]"
        # "256"
        # "256"
        # "4"
        # "256, 256, 4, 0"
        # "Parse: Shape wData\n(*)"
        n102 = Unbundle By Name(w292) -> ("nDim"=w297:i32[], "wData"=w290:sgl[])
        n103 = Index Array(array=w297) -> (element #1=w287:i32, element #2=w288:i32, element #3=w289:i32)  [unwired: 3 in]
        n104 = Initialize Array(sgl 0.0, w287, w288, w289) -> (w295:sgl[][][])
        n105 = for {
          N: w289 -> [_]
          tunnel: w288 -> [w308]
          tunnel: w287 -> [w307]
          shift-right: [w305] -> w286
          shift-left: w295 -> [w306]
          tunnel: w290 -> [w303]
          shift-right: [w301] -> _
          shift-left: 0 -> [w302]
          i -> [w304]
          n106 = for {
            N: w308 -> [_]
            tunnel: w307 -> [w316]
            shift-right: [w314] -> w305
            shift-left: w306 -> [w315]
            tunnel: w304 -> [w312]
            tunnel: w303 -> [w311]
            shift-right: [w309] -> w301
            shift-left: w302 -> [w310]
            i -> [w313]
            n107 = for {
              N: w316 -> [_]
              shift-right: [w324] -> w314
              shift-left: w315 -> [w325]
              tunnel: w313 -> [w322]
              tunnel: w312 -> [w321]
              tunnel: w311 -> [w320]
              shift-right: [w318] -> w309
              shift-left: w310 -> [w319]
              i -> [w323]
              n108 = Index Array(array=w320, index=w319) -> (element=w317:sgl)
              n109 = Replace Array Subset(array=w325, new element=w317, index (dim 0)=w323, index (dim 1)=w322, index (dim 2)=w321) -> (w324:sgl[][][])
              n110 = Increment(x=w319) -> (x+1=w318:i32)
            }
          }
        }
        n111 = Bundle By Name(cluster=w292, "wData"=sgl[] [], "Shaped wData"=w286) -> (w293:T5)
        n112 = call <vilib>:"Add State(s) to Queue__JKI_lib_State_Machine.vi"("State(s) in (\"\")"=w300) -> ("States Out"=w299:string)  [unwired: 14 in]
      }
      frame "Parse: Notes" {
        # "BinaryHeader5 size + wfmSize is the offset for the notes portion of the file."
        # "Parse: Notes\n(*)"
        n113 = Unbundle By Name(w327) -> ("Binary"=w333:string, "wfmSize"=w332:i32, "noteSize"=w329:i32)
        n114 = Add(x=w332, y=64) -> (x+y=w330:i32)
        n115 = String Subset(string=w333, offset (0)=w330, length (rest)=w329) -> (substring=w326:string)
        n116 = Bundle By Name(cluster=w327, "Notes"=w326) -> (w328:T5)
        n117 = call <vilib>:"Add State(s) to Queue__JKI_lib_State_Machine.vi"("State(s) in (\"\")"=w336) -> ("States Out"=w335:string)  [unwired: 14 in]
      }
      frame "---------- IMAQ ----------" {
        # "Template Separator\n(You can make a copy of, or modify, this frame)"
        n118 = call <vilib>:"Add State(s) to Queue__JKI_lib_State_Machine.vi"("State(s) in (\"\")"=w340) -> ("States Out"=w339:string)  [unwired: 14 in]
      }
      frame "IMAQ: Create" {
        # "Template Separator\n(You can make a copy of, or modify, this frame)"
        n119 = Unbundle By Name(w343) -> ("nDim"=w346:i32[], "Shaped wData"=w348:sgl[][][])
        n120 = Index Array(array=w346) -> (element #3=w347:i32)  [unwired: 3 in, 2 out]
        n121 = for {
          N: w347 -> [_]
          tunnel: [w363] -> w341 mode=indexing
          tunnel: w348 -> [w359]
          shift-right: [w356] -> w344
          shift-left: w345 -> [w354]
          tunnel: w342 -> [w351]
          i -> [w358]
          w353 = u32 0 items=["Horizontal", "Vertical", "Central", "1st Diagonal", "2nd Diagonal"] ("Type of Symmetry")
          w355 = T7 2 items=["Grayscale (U8)", "Grayscale (I16)", "Grayscale (SGL)", "Complex (CSG)", "RGB (U32)", "HSL (U32)", "RGB (U64)", "Grayscale (U16)"] ("Image Type")
          # "Flip to make it look right"
          # "Load array into IMAQ"
          # "Unique name for IMAQ Ref"
          n122 = Index Array(array=w359, index (dim 2)=w358) -> (element=w360:sgl[][])  [unwired: 2 in]
          n123 = Number To Decimal String(number=w358) -> (decimal integer string=w366:string)  [unwired: 1 in]
          n124 = Transpose 2D Array(2D array=w360) -> (transposed array=w357:sgl[][])
          n125 = Concatenate Strings(w351, w366) -> (w352:string)
          n126 = call "Imaq Create"("Image Name"=w352, "Image Type"=w355, "error in (no error)"=w354) -> ("New Image"=w365:T1, "error out"=w361:errorcluster)  [unwired: 1 in, 1 out]
          n127 = call "IMAQ ArrayToImage"("Image Pixels (Float)"=w357, "error in (no error)"=w361, "Image"=w365) -> ("error out"=w362:errorcluster, "Image Out"=w364:T1)  [unwired: 3 in, 4 out]
          n128 = call "IMAQ Symmetry"("error in (no error)"=w362, "Type of Symmetry"=w353, "Image Src"=w364) -> ("error out"=w356:errorcluster, "Image Dst Out"=w363:T1)  [unwired: 1 in, 1 out]
        }
        "IMAQ" <- w341
        n129 = call <vilib>:"Add State(s) to Queue__JKI_lib_State_Machine.vi"("State(s) in (\"\")"=w350) -> ("States Out"=w349:string)  [unwired: 14 in]
      }
      frame "---------- Notes ----------" {
        # "Template Separator\n(You can make a copy of, or modify, this frame)"
        n130 = call <vilib>:"Add State(s) to Queue__JKI_lib_State_Machine.vi"("State(s) in (\"\")"=w370) -> ("States Out"=w369:string)  [unwired: 14 in]
      }
      frame "Notes: Create LUT" {
        # "Notes: Create LUT\n(You can make a copy of, or modify, this frame)"
        n131 = Unbundle By Name(w378) -> ("Notes"=w377:string)
        n132 = call <vilib>:"Delimited String to 1D String Array.vi"("delimiter"="\r" ("Carriage Return Constant"), "delimited string"=w377) -> ("string array"=w376:string[])  [unwired: 9 in]
        n133 = for {
          tunnel: w376 -> [w391] mode=indexing
          shift-right: [w387] -> w373
          shift-left: variant -> [w386]
          shift-right: [w383] -> w372
          shift-left: w371 -> [w384]
          w388 = T8 1 items=["both", "start of string", "end of string"] ("location (both)")
          # "If the line is empty, dont write it to LUT"
          n134 = Match Pattern(string=w391, regular expression="\\:") -> (before substring=w382:string, after substring=w389:string)  [unwired: 1 in, 2 out]
          n135 = call <vilib>:"Trim Whitespace.vi"("string"=w389, "location (both)"=w388) -> ("trimmed string"=w381:string)
          n136 = Empty String/Path?(string/path=w382) -> (empty?=w385:bool)
          n137 = case shown="False" w385 {
            tunnel: [w397 w399] -> w387
            tunnel: w386 -> [w396 w399]
            tunnel: w381 -> [w395 _]
            tunnel: w382 -> [w394 _]
            tunnel: w384 -> [w393 w398]
            tunnel: [w392 w398] -> w383
            frame False {
              n138 = Set Variant Attribute(Variant=w396, name=w394, value=w395, error in=w393) -> (Variant out=w397:variant, error out=w392:errorcluster)  [unwired: 1 out]
            }
            frame True {
            }
          }
        }
        "Notes LUT" <- w373
        n139 = call <vilib>:"Add State(s) to Queue__JKI_lib_State_Machine.vi"("State(s) in (\"\")"=w380) -> ("States Out"=w379:string)  [unwired: 14 in]
      }
      frame "---------- Directory ----------" {
        # "Template Separator\n(You can make a copy of, or modify, this frame)"
        n140 = call <vilib>:"Add State(s) to Queue__JKI_lib_State_Machine.vi"("State(s) in (\"\")"=w403) -> ("States Out"=w402:string)  [unwired: 14 in]
      }
      frame "Directory: Bin Header" {
        # "This is a key for the string lengths and Indices of all of the values in the bin header"
        # "Length|Index|typedef struct BinHeader5 {\n     2|    0|\tshort version;\t\t\t\t\t\t          // Version number for backwards compatibility.\n     2|    2|\tshort checksum;\t\t\t\t\t\t         // Checksum over this header and the wave header.\n     4|    4|\tlong wfmSize;\t\t\t\t\t\t           // The size of the WaveHeader5 data structure plus the wave data.\n     4|    8|\tlong formulaSize;\t\t\t\t\t        // The size of the dependency formula, if any.\n     4|   12|\tlong noteSize;\t\t\t\t\t\t          // The size of the note text.\n     4|   16|\tlong dataEUnitsSize;\t\t\t\t      // The size of optional extended data units.\n    16|   20|\tlong dimEUnitsSize[MAXDIMS];\t\t// The size of optional extended dimension units.\n    16|   36|\tlong dimLabelsSize[MAXDIMS];\t\t// The size of optional dimension labels.\n     4|   52|\tlong sIndicesSize;\t\t\t\t\t       // The size of string indicies if this is a text wave.\n     4|   56|\tlong optionsSize1;\t\t\t\t\t       // Reserved. Write zero. Ignore on read.\n     4|   60|\tlong optionsSize2;\t\t\t\t\t       // Reserved. Write zero. Ignore on read.\n      |   64|} BinHeader5;"
        n141 = call <vilib>:"Add State(s) to Queue__JKI_lib_State_Machine.vi"("State(s) in (\"\")"=w407) -> ("States Out"=w406:string)  [unwired: 14 in]
      }
      frame "Directory: Wave Header" {
        # "Expand to see all documentation"
        # "Length|Index|struct WaveHeader5 {\n     4|   64|\tstruct WaveHeader5 **next;\t\t\t  // link to next wave in linked list.\n     4|   68|\tunsigned long creationDate;\t\t \t// DateTime of creation.\n     4|   72|\tunsigned long modDate;\t\t\t\t     // DateTime of last modification.\n     4|   76|\tlong npnts;\t\t\t\t\t\t\t             // Total number of points (multiply dimensions up to first zero).\n     2|   80|\tshort type;\t\t\t\t\t\t\t             // See types (e.g. NT_FP64) above. Zero for text waves.\n     2|   82|\tshort dLock;\t\t\t\t\t\t             // Reserved. Write zero. Ignore on read.\n     6|   84|\tchar whpad1[6];\t\t\t\t\t\t          // Reserved. Write zero. Ignore on read.\n     2|   90|\tshort whVersion;\t\t\t\t\t          // Write 1. Ignore on read.\n    32|   92|\tchar bname[MAX_WAVE_NAME5+1];\t\t// Name of wave plus trailing null.\n     4|  124|\tlong whpad2;\t\t\t\t\t\t             // Reserved. Write zero. Ignore on read.\n     4|  128|\tstruct DataFolder **dFolder;\t\t // Used in memory only. Write zero. Ignore on read.\n      |     |\t// Dimensioning info. [0] == rows, [1] == cols etc\n    16|  132|\tlong nDim[MAXDIMS];\t\t\t\t\t       // Number of of items in a dimension -- 0 means no data.\n    32|  148|\tdouble sfA[MAXDIMS];\t\t\t\t       // Index value for element e of dimension d = sfA[d]*e + sfB[d].\n    32|  180|\tdouble sfB[MAXDIMS];\n      |     |\t// SI units\n     4|  212|\tchar dataUnits[MAX_UNIT_CHARS+1];\t\t\t      // Natural data units go here - null if none.\n    16|  216|\tchar dimUnits[MAXDIMS][MAX_UNIT_CHARS+1];\t// Natural dimension units go here - null if none.\n     2|  232|\tshort fsValid;\t\t\t\t\t\t                      // TRUE if full scale values have meaning.\n     2|  234|\tshort whpad3;\t\t\t\t\t\t                       // Reserved. Write zero. Ignore on read.\n    16|  236|\tdouble topFullScale,botFullScale;\t        // The max and max full scale value for wave.\n     4|  252|\tHandle dataEUnits;\t\t\t\t\t                   // Used in memory only. Write zero. Ignore on read.\n    16|  256|\tHandle dimEUnits[MAXDIMS];\t\t\t             // Used in memory only. Write zero. Ignore on read.\n    16|  272|\tHandle dimLabels[MAXDIMS];\t\t\t             // Used in memory only. Write zero. Ignore on read.\n     4|  288|\tHandle waveNoteH;\t\t\t\t\t                    // Used in memory only. Write zero. Ignore on read.\n    64|  292|\tlong whUnused[16];\t\t\t\t\t                   // Reserved. Write zero. Ignore on read.\n      |     |\t// The following stuff is considered private to Igor.\n     2|  356|\tshort aModified;\t\t\t\t\t                     // Used in memory only. Write zero. Ignore on read.\n     2|  358|\tshort wModified;\t\t\t\t\t                     // Used in memory only. Write zero. Ignore on read.\n     2|  360|\tshort swModified;\t\t\t\t\t                    // Used in memory only. Write zero. Ignore on read.\n     1|  362|\tchar useBits;\t\t\t\t\t\t                       // Used in memory only. Write zero. Ignore on read.\n     1|  363|\tchar kindBits;\t\t\t\t\t\t                      // Reserved. Write zero. Ignore on read.\n     4|  364|\tvoid **formula;\t\t\t\t\t\t                     // Used in memory only. Write zero. Ignore on read.\n     4|  368|\tlong depID;\t\t\t\t\t\t\t                        // Used in memory only. Write zero. Ignore on read.\n     2|  372|\tshort whpad4;\t\t\t\t\t\t                       // Reserved. Write zero. Ignore on read.\n     2|  374|\tshort srcFldr;\t\t\t\t\t\t                      // Used in memory only. Write zero. Ignore on read.\n     4|  376|\tHandle fileName;\t\t\t\t\t                     // Used in memory only. Write zero. Ignore on read.\n     4|  380|\tlong **sIndices;\t\t\t\t\t                     // Used in memory only. Write zero. Ignore on read.\n     4|  384|\tfloat wData[1];\t\t\t\t\t\t                     // The start of the array of data. Must be 64 bit aligned.\n      |  388|};"
        # "This is a key for the string lengths and Indices of all of the values in the wave header"
        n142 = call <vilib>:"Add State(s) to Queue__JKI_lib_State_Machine.vi"("State(s) in (\"\")"=w411) -> ("States Out"=w410:string)  [unwired: 14 in]
      }
    }
  }
  "error out" <- w3
